vi "BoxcarFilter.vi"(8 "error in (no error)":errorcluster, 10 "Half Width":i32, 11 "Signal":dynamicdata(graph)) -> (0 "error out":errorcluster, 3 "Filtered Signal":dynamicdata(graph))   [LabVIEW 2013]
doc: "Processes signals through filters and windows.\n--------------------\n\nThis Express VI is configured as follows:\n\nFilter Type: Smoothing"
panel:
  out "Signals In":dynamicdata(graph)
  in  "Upper Cut-Off":dbl=400.0
  in  "Lower Cut-Off":dbl=100.0
  in  "Order":u32=3
  in  "Filter Type":u16(ring)=4 items=["Lowpass", "Highpass", "Bandpass", "Bandstop"]
  in  "Filter Topology":u16(ring)=1 items=["Off", "Butterworth", "Chebyshev", "Inverse Chebyshev", "Elliptic", "Bessel"]
  in  "#Taps":u32=29
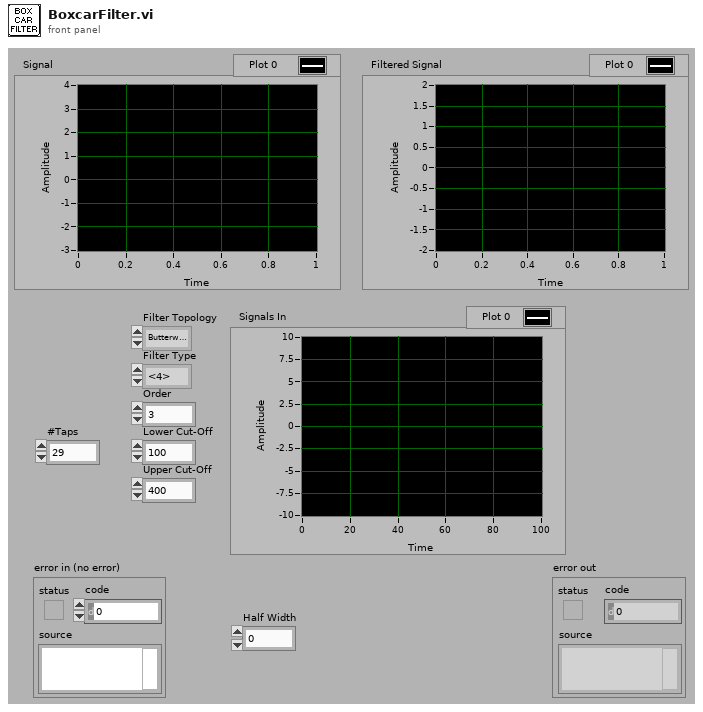
[diagram p1: front panel]
types:
  T1 = cluster{"half-width of moving average":i32, "smoothing filter type":u16, "shape of moving averager":u16, "time constant of exponential average":dbl}
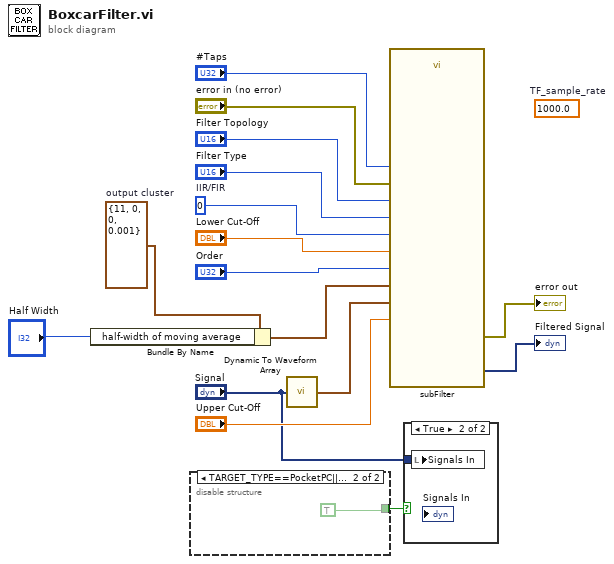
[diagram p0: block diagram]
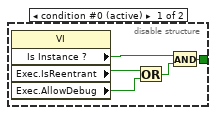
[diagram p2: hidden frame]
diagram:
  w3 = T1 {"half-width of moving average"=11, "smoothing filter type"=0, "shape of moving averager"=0, "time constant of exponential average"=0.001}  # output cluster
  (unwired) 1000.0  # TF_sample_rate
  w14 = 0  # IIR/FIR
  n1 = Bundle By Name(cluster=w3, "half-width of moving average"="Half Width") -> (w2:T1)
  n2 = disable-structure shown="TARGET_TYPE==PocketPC||TARGET_TYPE==PalmOS||TARGET_TYPE==Embedded" {
    disable-tunnel: [w21 TRUE] -> w5
    frame condition #0 (active) {
      n3 = property class="VI"() -> ("Is Instance ?"=w20:bool, "Exec.IsReentrant"=w18:bool, "Exec.AllowDebug"=w17:bool)  [unwired: 2 in, 2 out]
      n4 = Or(x=w18, y=w17) -> (x .or. y?=w19:bool)
      n5 = And(x=w20, y=w19) -> (x .and. y?=w21:bool)
    }
    frame condition #1 {
    }
  }
  n6 = call <vilib>:"Dynamic To Waveform Array.vi"("Input"="Signal") -> ("Output"=w16:waveform(dbl)[])  [unwired: 4 in]
  n7 = call <vilib>:"subFilter.vi"("Signals"=w16, "Filter Type"="Filter Type", "#Taps"="#Taps", "IIR/FIR"=w14, "Lower Cut-Off"="Lower Cut-Off", "Upper Cut-Off"="Upper Cut-Off", "error in (no error)"="error in (no error)", "Filter Topology"="Filter Topology", "Order"="Order", "output cluster"=w2) -> ("Filtered Signals"=→"Filtered Signal":dynamicdata, "error out"=→"error out":errorcluster)  [unwired: 3 in, 1 out]
  n8 = case shown="True" w5 {
    tunnel: "Signal" -> [_ w23]
    frame False {
    }
    frame True {
      n9 = local write "Signals In"(w23) -> ()
    }
  }
